vi "LbcbConversionsFactory.vi"(8 "error in (no error)":errorcluster, 9 "LbcbConversionType":T1, 10 "LBCB Number":T2, 11 "Actions":T3) -> (0 "error out":errorcluster, 2 "Conversion Ref":refnum<k24>)   [LabVIEW 2013]
uses:
  Data Access Objects/Metadata/DAO Actions with Remove.ctl
  Data Access Objects/Metadata/LBCB Number.ctl
  LbcbConversionTypes.ctl
  C:/Users/mbletzin/Desktop/Work/OM/DLL/LbcbConversions.dll
  DLL/LbcbConversions.dll
  Data Access Objects/Metadata/Persistant DAO Actions.ctl
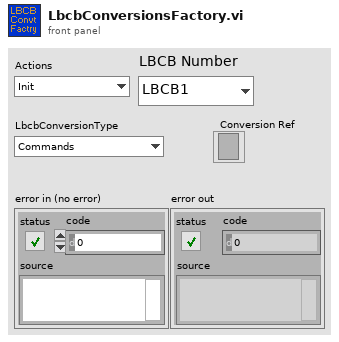
[diagram p1: front panel]
types:
  T1 = typedef "LbcbConversionTypes.ctl" = enum16{"Commands", "Readings", "Offsets"}
  T2 = typedef "LBCB Number.ctl" = enum16{"LBCB1", "LBCB2"}
  T3 = typedef "DAO Actions with Remove.ctl" = enum16{"Init", "Get", "Set", "Remove"}
  T4 = typedef "Persistant DAO Actions.ctl" = enum16{"Init", "Get", "Set", "Load", "Save"}
  T5 = typedef "LBCB Position.ctl" = cluster{"Motion Center":dbl[], "Transformation Matrix":dbl[][]}
  T6 = typedef "LBCB Pin Positions.ctl" = cluster{"Pin Positions":dbl[][]}
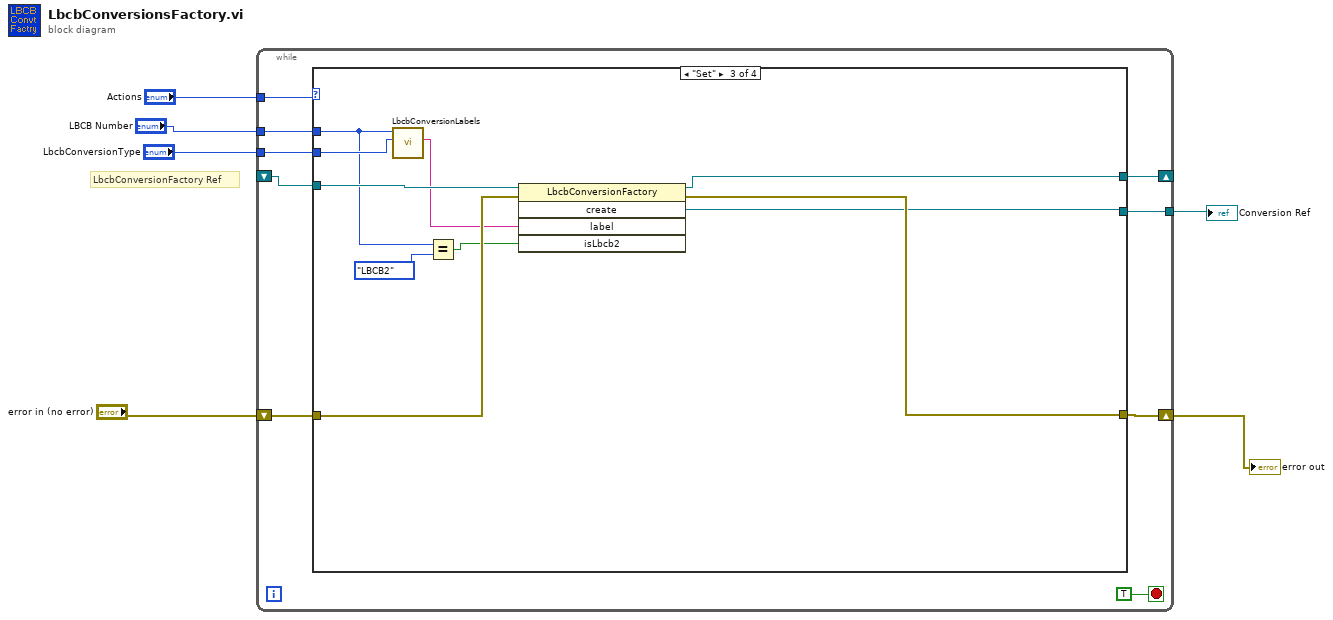
[diagram p0: block diagram]
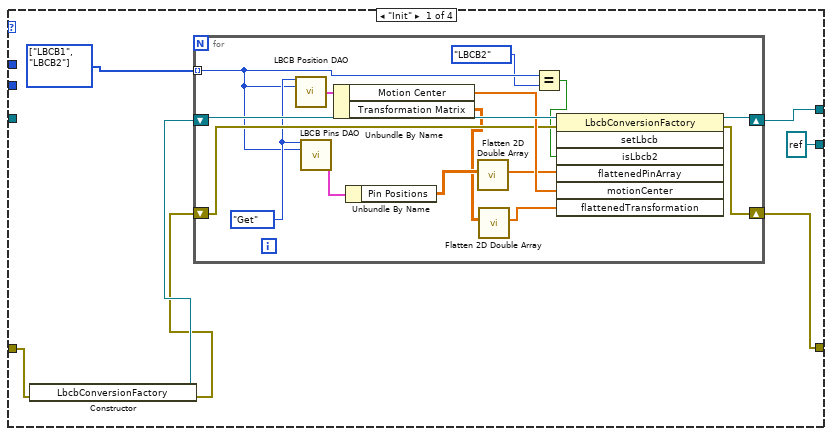
[diagram p2: hidden frame]
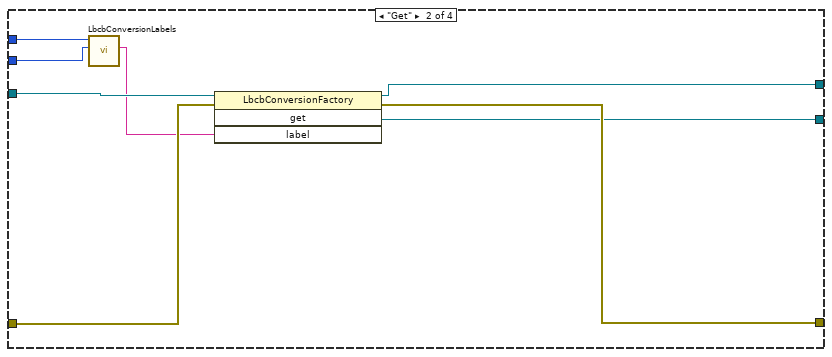
[diagram p3: hidden frame]
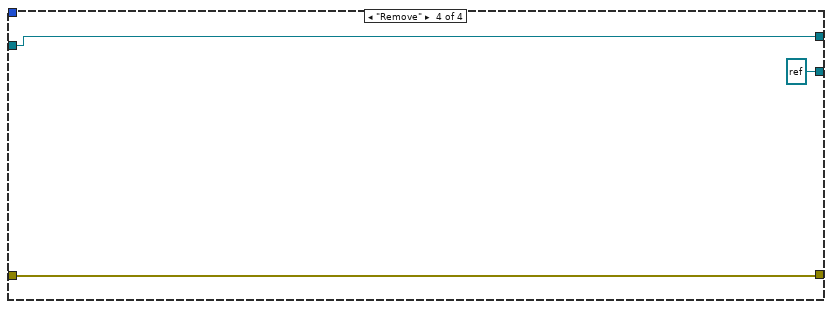
[diagram p4: hidden frame]
diagram:
  # "LbcbConversionFactory Ref"
  n1 = while {
    tunnel: "Actions" -> [w14]
    shift-right: [w12] -> w4
    shift-left: "error in (no error)" -> [w13]
    shift-right: [w11] -> _
    shift-left: _ -> [w10]
    tunnel: "LBCB Number" -> [w9]
    tunnel: "LbcbConversionType" -> [w8]
    tunnel: [w7] -> w1
    stop <- TRUE stop-if-true
    n2 = case shown="\"Set\"" w14 {
      tunnel: w13 -> [w22 w44 w54 w58]
      tunnel: [w19 w39 w50 w58] -> w12
      tunnel: [w17 w43 w53 w57] -> w11
      tunnel: w10 -> [_ w45 w55 w57]
      tunnel: w9 -> [_ w42 w49 _]
      tunnel: w8 -> [_ w41 w52 _]
      tunnel: [refnum<k24> refnum ("create") w38 w46 refnum<k24> refnum ("create")] -> w7
      frame "Init" {
        w18 = T2[] [enum."LBCB1", enum."LBCB2"] items=["LBCB1", "LBCB2"]
        n3 = constructor class="LbcbConversionFactory"(error in=w22) -> (reference out=w21:refnum<k24>, error out=w20:errorcluster)  [unwired: 2 in, 1 out]
        n4 = for {
          tunnel: w18 -> [w27] mode=indexing
          shift-right: [w33] -> w19
          shift-left: w20 -> [w34]
          shift-right: [w25] -> w17
          shift-left: w21 -> [w37]
          w32 = Persistant_DAO_Actions."Get" ("LBCB Settings Actions")
          n5 = call "LBCB Position DAO.vi"("LBCB Settings Actions"=w32, "LBCB Number"=w27) -> ("LBCB Position Output"=w36:T5)  [unwired: 11 in, 2 out]
          n6 = call "LBCB Pins DAO.vi"("LBCB Settings Actions"=w32, "LBCB Number"=w27) -> ("LBCB Pins Output"=w31:T6)  [unwired: 11 in, 2 out]
          n7 = Unbundle By Name(w36) -> ("Motion Center"=w35:dbl[], "Transformation Matrix"=w24:dbl[][])
          n8 = Unbundle By Name(w31) -> ("Pin Positions"=w30:dbl[][])
          n9 = call "Flatten 2D Double Array.vi"("Input Double Matrix"=w30) -> ("Flattened Array"=w29:dbl[])  [unwired: 10 in]
          n10 = call "Flatten 2D Double Array.vi"("Input Double Matrix"=w24) -> ("Flattened Array"=w23:dbl[])  [unwired: 10 in]
          n11 = Equal?(x=w27, y=LBCB_Number."LBCB2") -> (x = y?=w28:bool)
          n12 = invoke class="LbcbConversionFactory" method="setLbcb"(reference=w37, error in=w34, "isLbcb2"=w28, "flattenedPinArray"=w29, "motionCenter"=w35, "flattenedTransformation"=w23) -> (reference out=w25:refnum<k24>, error out=w33:errorcluster)  [unwired: 1 in, 5 out]
        }
      }
      frame "Get" {
        n13 = call "LbcbConversionLabels.vi"("LbcbConversionType"=w41, "LBCB Number"=w42) -> ("Conversion Label"=w40:string)  [unwired: 9 in]
        n14 = invoke class="LbcbConversionFactory" method="get"(reference=w45, error in=w44, "label"=w40) -> (reference out=w43:refnum<k24>, error out=w39:errorcluster, "get"=w38:refnum<k24>)  [unwired: 1 in, 1 out]
      }
      frame "Set" {
        n15 = call "LbcbConversionLabels.vi"("LbcbConversionType"=w52, "LBCB Number"=w49) -> ("Conversion Label"=w51:string)  [unwired: 9 in]
        n16 = Equal?(x=w49, y=LBCB_Number."LBCB2") -> (x = y?=w47:bool)
        n17 = invoke class="LbcbConversionFactory" method="create"(reference=w55, error in=w54, "label"=w51, "isLbcb2"=w47) -> (reference out=w53:refnum<k24>, error out=w50:errorcluster, "create"=w46:refnum<k24>)  [unwired: 1 in, 2 out]
      }
      frame "Remove" {
      }
    }
  }
  "error out" <- w4
  "Conversion Ref" <- w1
